vi "TriggerDelay.vi"(10 "Delay":u32, 11 "In":bool) -> (2 "Off":bool, 3 "Out":bool)   [LabVIEW 2012]
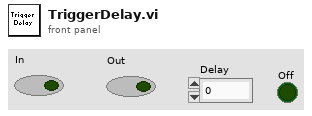
[diagram p1: front panel]
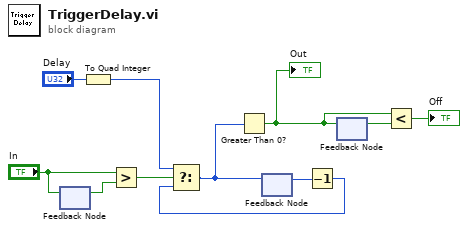
[diagram p0: block diagram]
diagram:
  n1 = feedback-in #1("In") -> ()
  n2 = feedback #1() -> (w10:bool)  [unwired: 1 in]
  n3 = To Quad Integer(1:"Delay") -> (0:w5:i64)
  n4 = Greater?(x="In", y=w10) -> (0:w9:bool)
  n5 = feedback #2() -> (w8:i64)  [unwired: 1 in]
  n6 = Decrement(x=w8) -> (x-1=w7:i64)
  n7 = Select(t=w5, s=w9, f=w7) -> (s? t:f=w4:i64)
  n8 = Greater Than 0?(x=w4) -> (x > 0?=w3:bool)
  "Out" <- w3
  n9 = feedback-in #2(w4) -> ()
  n10 = feedback #3() -> (w2:bool)  [unwired: 1 in]
  n11 = feedback-in #3(w3) -> ()
  n12 = Less?(x=w3, y=w2) -> (x < y?=→"Off":bool)
